vi "Init.vi"(8 "error in (no error)":errorcluster, 9 "Trigger Config In":variant, 10 "DIO Config In":variant, 11 "DIO in":refnum<class "DIO.lvclass">) -> (0 "error out":errorcluster, 3 "DIO out":refnum<class "DIO.lvclass">)   [LabVIEW 2015, in "DIO.lvclass"]
uses:
  DIO.lvclass
  DIO.lvclass/DIO.ctl
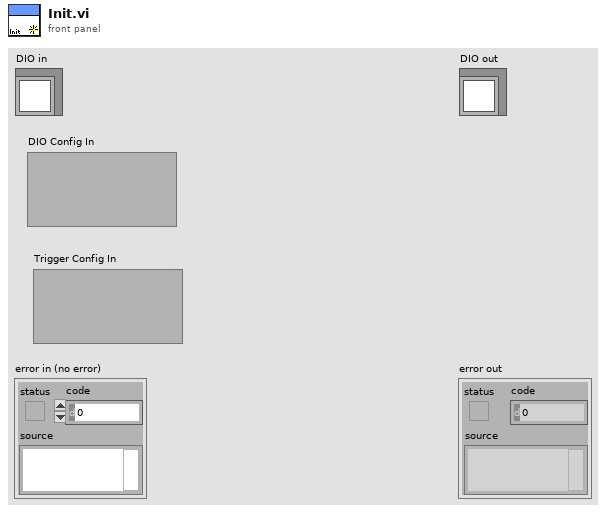
[diagram p1: front panel]
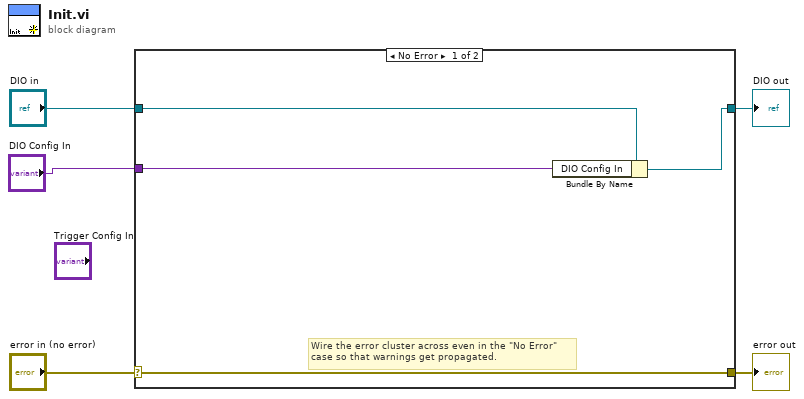
[diagram p0: block diagram]
diagram:
  n1 = case shown="No Error" "error in (no error)" {
    selector: "error in (no error)" -> [w9 w11]
    tunnel: [w9 w11] -> w4
    tunnel: [w7 w10] -> w2
    tunnel: "DIO in" -> [w8 w10]
    tunnel: "DIO Config In" -> [w6 _]
    frame No Error {
      # "Wire the error cluster across even in the \"No Error\"\ncase so that warnings get propagated."
      n2 = Bundle By Name(cluster=w8, "DIO Config In"=w6) -> (w7:refnum<class "DIO.lvclass">)
    }
    frame Error {
    }
  }
  "error out" <- w4
  "DIO out" <- w2
